vi "DisConnect.vi"(8 "error in (no error)":errorcluster, 11 "Red Pitaya in":refnum<class "Red Pitaya.lvclass">) -> (0 "error out":errorcluster, 3 "Red Pitaya out":refnum<class "Red Pitaya.lvclass">)   [LabVIEW 2015, in "Red Pitaya.lvclass"]
uses:
  Red Pitaya.lvclass
  NHMFL_Core/Libraries/Red Pitaya/RP Command.ctl
  Red Pitaya.lvclass/Red Pitaya.ctl
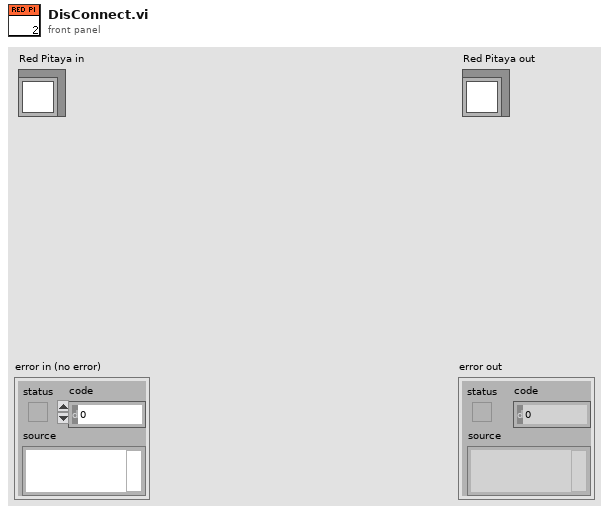
[diagram p1: front panel]
types:
  T1 = typedef "RP Command.ctl" = enum16{"Set frequency", "Arm and get data", "Stop server", "Get status", "Get temperature", "Set decimation", "Arm", "Software trigger", "Get whole buffer", "Get chunk", "System call", "Get config", "Set config", "Read FIFO", "Play pattern", "Set frequency batch"}
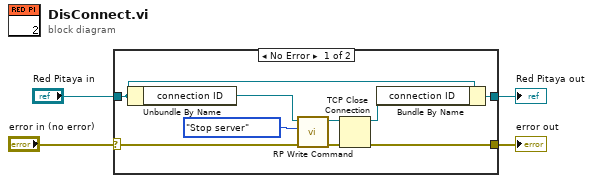
[diagram p0: block diagram]
diagram:
  n1 = case shown="No Error" "error in (no error)" {
    selector: "error in (no error)" -> [w5 w15]
    tunnel: [w10 w15] -> w3
    tunnel: [w12 w14] -> w1
    tunnel: "Red Pitaya in" -> [w13 w14]
    frame No Error {
      n2 = Unbundle By Name(w13) -> ("connection ID"=w7:refnum<k5>)
      n3 = call "RP Write Command.vi"("Error In"=w5, "Command number"=RP_Command."Stop server", "connection ID"=w7) -> ("Error Out"=w6:errorcluster, "connection ID out"=w8:refnum<k5>)  [unwired: 6 in, 1 out]
      n4 = TCP Close Connection(connection ID=w8, error in (no error)=w6) -> (connection ID out=w11:refnum<k5>, error out=w10:errorcluster)  [unwired: 1 in]
      n5 = Bundle By Name(cluster=w13, "connection ID"=w11) -> (w12:refnum<class "Red Pitaya.lvclass">)
    }
    frame Error {
    }
  }
  "error out" <- w3
  "Red Pitaya out" <- w1
